vi "Read Measurement (Voltage).vi"(6 "Wait Time (10 S)":i32=10, 8 "error in (no error)":errorcluster, 9 "Voltage Buffer (smua.nvbuffer1)":string="smua.nvbuffer1", 10 "Source Measure Unit Channel (0: Channel A)":i32(ring) items=["Channel A", "Channel B"], 11 "VISA resource name":refnum<visa-resource-name>) -> (0 "error out":errorcluster, 1 "Last Voltage (V)":dbl, 3 "VISA resource name out":refnum<visa-resource-name>, 4 "Voltage Buffer Data (V)":dbl[](array[numeric]))   [LabVIEW 2020, in "Keithley 2600 Series.lvlib"]
doc: "Returns the measured voltage."
uses:
  <instrlib>/Keithley 2600 Series/Keithley 2600 Series.lvlib
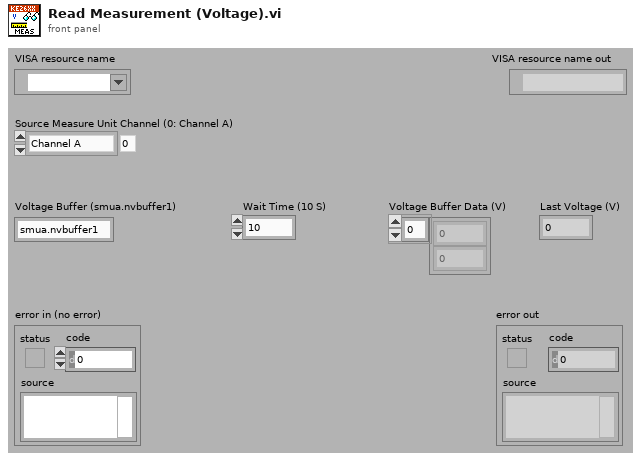
[diagram p1: front panel]
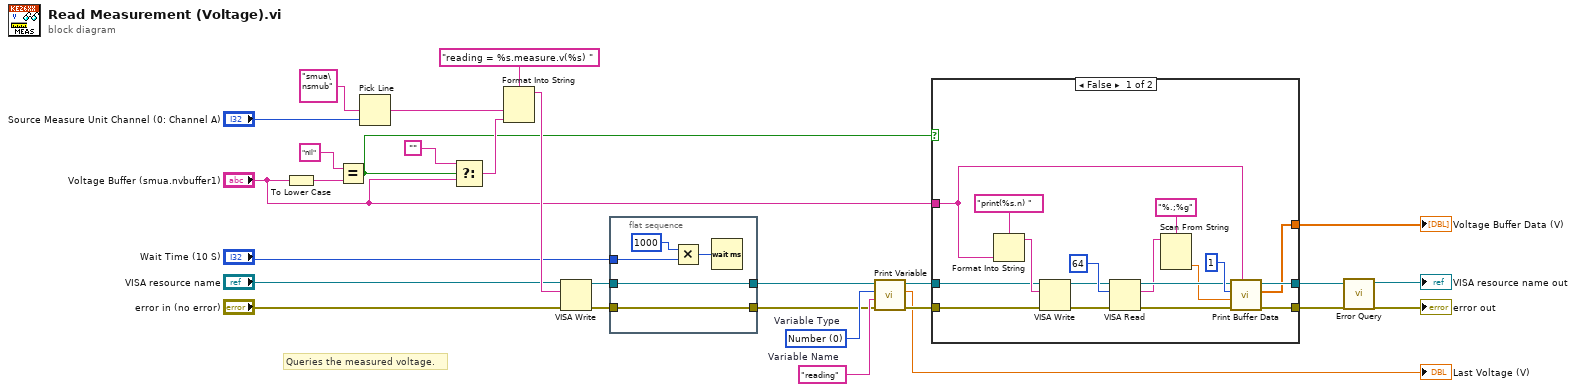
[diagram p0: block diagram]
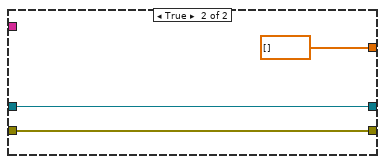
[diagram p2: hidden frame]
diagram:
  w7 = "reading"  # Variable Name
  w8 = 0 items=["Number", "Message"]  # Variable Type
  # "Queries the measured voltage."
  n1 = To Lower Case(string="Voltage Buffer (smua.nvbuffer1)") -> (all lower case string=w9:string)
  n2 = Equal?(x="nil", y=w9) -> (x = y?=w20:bool)
  n3 = Pick Line(multi-line string="smua\nsmub", line index="Source Measure Unit Channel (0: Channel A)") -> (output string=w24:string)  [unwired: 1 in]
  n4 = Select(t="", s=w20, f="Voltage Buffer (smua.nvbuffer1)") -> (s? t:f=w21:string)
  n5 = Format Into String(format string="reading = %s.measure.v(%s) ", w24, w21) -> (resulting string=w26:string)  [unwired: 2 in, 1 out]
  n6 = VISA Write(VISA resource name="VISA resource name", write buffer=w26, error in (no error)="error in (no error)") -> (VISA resource name out=w19:refnum<visa-resource-name>, error out=w18:errorcluster)  [unwired: 1 out]
  n7 = flat-sequence {
    tunnel: w19 -> [w33]
    tunnel: [w33] -> w4
    tunnel: w18 -> [w32]
    tunnel: [w32] -> w3
    tunnel: "Wait Time (10 S)" -> [w29]
    frame #0 {
      n8 = Multiply(x=1000 ("y"), y=w29) -> (x*y=w31:i32)
      n9 = Wait (ms)(milliseconds to wait=w31) -> ()  [unwired: 1 out]
    }
  }
  n10 = call <instrlib>:"Print Variable.vi"("error in (no error)"=w3, "Variable Name"=w7, "Variable Type (0: Number)"=w8, "VISA resource name"=w4) -> ("error out"=w5:errorcluster, "Number"=→"Last Voltage (V)":dbl, "VISA resource name out"=w6:refnum<visa-resource-name>)  [unwired: 4 in, 1 out]
  n11 = case shown="False" w20 {
    tunnel: w6 -> [w39 w53]
    tunnel: w5 -> [w38 w52]
    tunnel: [w37 w53] -> w11
    tunnel: [w36 w52] -> w10
    tunnel: [w35 dbl[] [] ("Buffer Data")] -> w12
    tunnel: "Voltage Buffer (smua.nvbuffer1)" -> [w34 _]
    frame False {
      n12 = Format Into String(format string="print(%s.n) ", w34) -> (resulting string=w40:string)  [unwired: 2 in, 1 out]
      n13 = VISA Write(VISA resource name=w39, write buffer=w40, error in (no error)=w38) -> (VISA resource name out=w43:refnum<visa-resource-name>, error out=w42:errorcluster)  [unwired: 1 out]
      n14 = VISA Read(VISA resource name=w43, byte count=u32 64, error in (no error)=w42) -> (VISA resource name out=w48:refnum<visa-resource-name>, read buffer=w46:string, error out=w47:errorcluster)  [unwired: 1 out]
      n15 = Scan From String(format string="%.;%g", input string=w46) -> (output 1=w45:dbl)  [unwired: 3 in, 3 out]
      n16 = call <instrlib>:"Print Buffer Data.vi"("Reading Buffer (smua.nvbuffer1)"=w34, "error in (no error)"=w47, "End Index (1)"=w45, "Start Index (1)"=1 ("Start Index (0)"), "VISA resource name"=w48) -> ("error out"=w36:errorcluster, "Buffer Data"=w35:dbl[], "VISA resource name out"=w37:refnum<visa-resource-name>)  [unwired: 4 in]
    }
    frame True {
    }
  }
  "Voltage Buffer Data (V)" <- w12
  n17 = call <instrlib>:"Error Query.vi"("error in (no error)"=w10, "VISA resource name"=w11) -> ("error out"=→"error out":errorcluster, "VISA resource name out"=→"VISA resource name out":refnum<visa-resource-name>)  [unwired: 6 in, 2 out]
